vi "V3test.vi"() -> ()   [LabVIEW 2019]
uses:
  WSCbot_V3_Toolkit.lvlibp/WSCBOTV3_Toolkit/Sensor/LowLevel/IR_Chanel.ctl
  WSCbot_V3_Toolkit.lvlibp/WSCBOTV3_Toolkit/MotorControl/LowLevel/ZRaxisRotatingSet.vi
  WSCbot_V3_Toolkit.lvlibp/WSCBOTV3_Toolkit/MotorControl/LowLevel/ZaxisSlideSet.vi
  WSCbot_V3_Toolkit.lvlibp/WSCBOTV3_Toolkit/Sensor/LowLevel/InfraredRanging(Array).vi
  WSCbot_V3_Toolkit.lvlibp
panel:
  in  "?":T1(tab)
  out "EMS":bool
  in  "蜂鳴器":bool
  out "步進馬達旋轉歸零":bool
  out "步進馬達上下歸零":bool
  in  "LED":bool
  in  "旋轉測試":bool
  in  "上下測試":bool
  in  "Enable_R":bool=TRUE
  in  "Enable_L":bool=TRUE
  out "Distance_L(mm)":dbl
  out "Distance_R(mm)":dbl
  out "Valtage":dbl[](array[numeric])
  in  "IR_Chanel":T2[](array[typedef])
  out "R":dbl(graph)
  out "L":dbl(graph)
  in  "Wheel":u16(ring) items=["127mm", "150mm", "100mm"]
  in  "底盤馬達測試":bool
  in  "Speed/ACC":cluster{dbl, dbl}={1000.0, 1000.0}
  in  "XYZ":cluster{"X":dbl, "Y":dbl, "Z":dbl}[](array[cluster])=[{"X"=0.0, "Y"=0.0, "Z"=0.0}]
  in  "Enable?":bool=TRUE
  in  "底盤馬達測試":bool
  in  "4xMotor(deg/s)":dbl[](array[numeric])=[0.0, 0.0, 0.0, 0.0]
  out "ENC (deg)":dbl[](array[numeric])
  out "ENC (deg)":dbl[](array[numeric])
  in  "Stop Button":bool
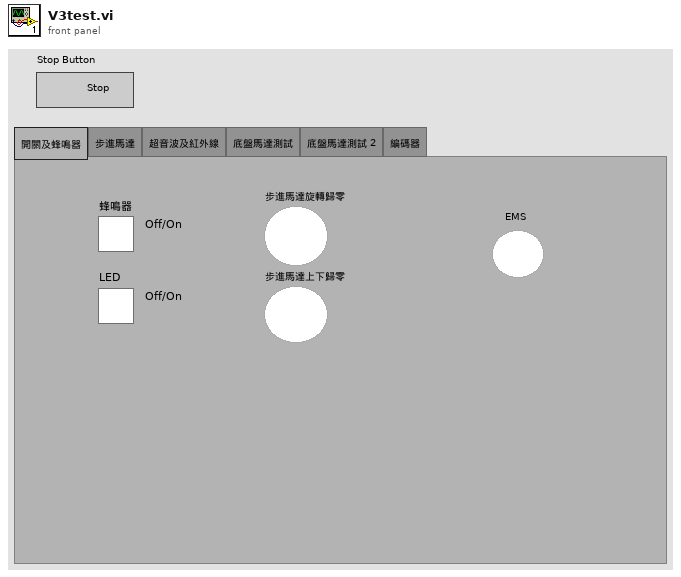
[diagram p1: front panel]
types:
  T1 = enum32{"開關及蜂鳴器", "步進馬達", "超音波及紅外線", "底盤馬達測試", "底盤馬達測試 2", "編碼器"}
  T2 = typedef "WSCbot_V3_Toolkit.lvlibp/IR_Chanel.ctl" = enum16{"IR_LF", "IR_LB", "IR_BL", "IR_BR", "IR_RB", "IR_RF", "IR_FR", "IR_FL"}
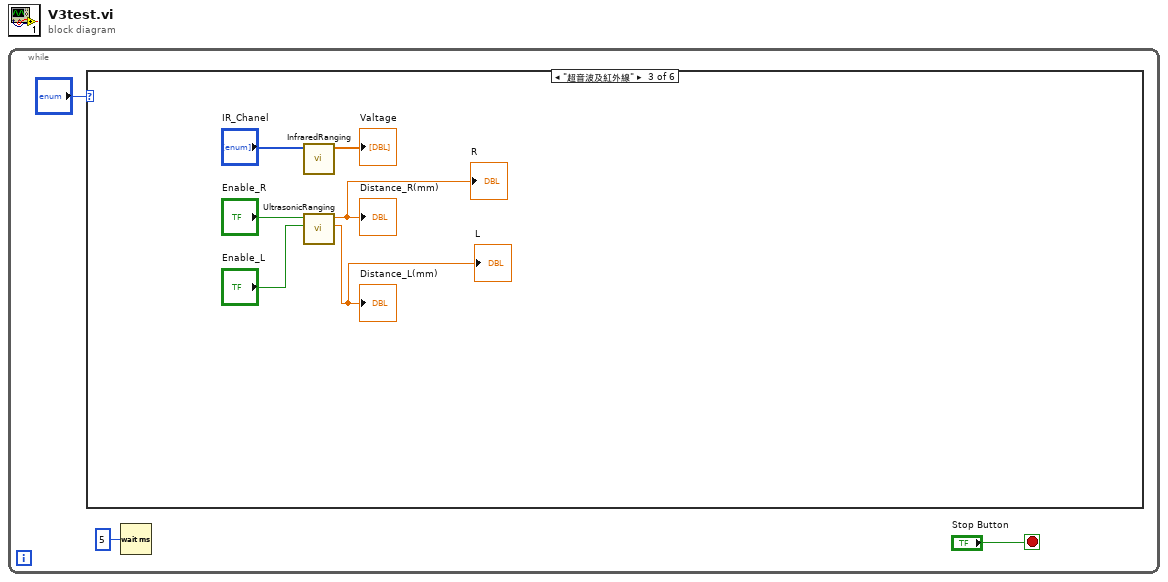
[diagram p0: block diagram]
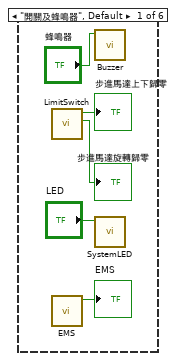
[diagram p2: hidden frame]
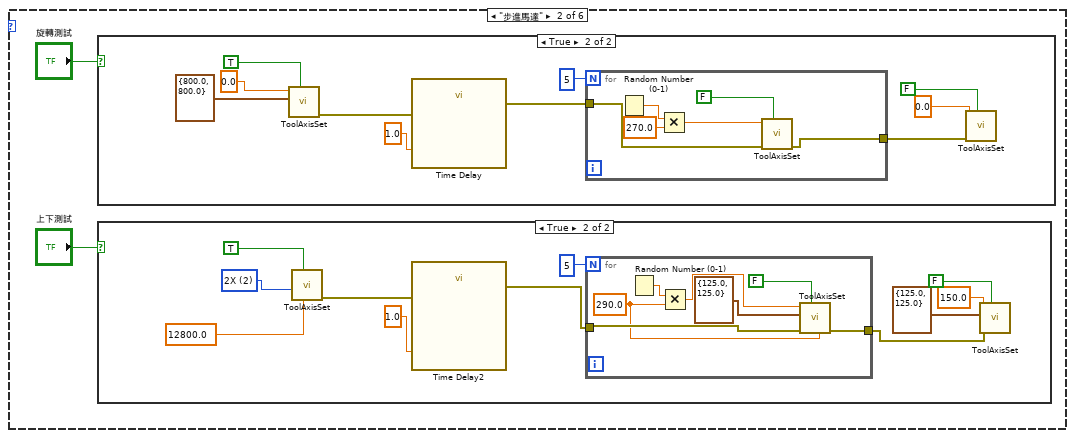
[diagram p3: hidden frame]
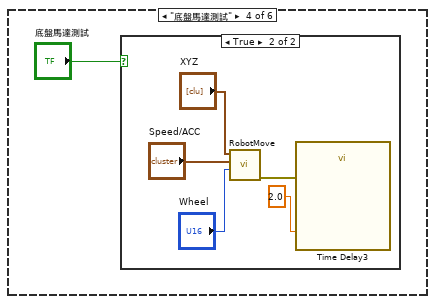
[diagram p6: hidden frame]
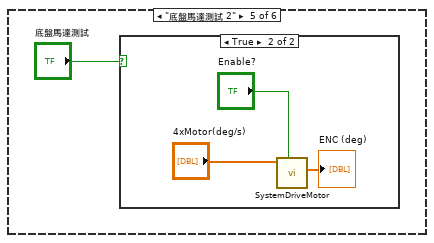
[diagram p8: hidden frame]
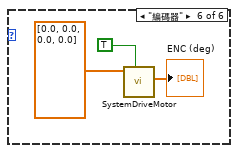
[diagram p10: hidden frame]
diagram:
  n1 = while {
    stop <- "Stop Button" stop-if-true
    n2 = case shown="\"超音波及紅外線\"" "?" {
      frame "開關及蜂鳴器", Default {
        n3 = call "LimitSwitch.vi"() -> ("LS11_ZR_IN"=→"步進馬達旋轉歸零":bool, "LS11_Z_IN"=→"步進馬達上下歸零":bool)  [unwired: 9 in, 1 out]
        n4 = call "EMS.vi"() -> ("EMS"=→"EMS":bool)  [unwired: 10 in, 1 out]
        n5 = call "Buzzer.vi"("Set"="蜂鳴器") -> ()  [unwired: 10 in, 1 out]
        n6 = call "SystemLED.vi"("Set"="LED") -> ()  [unwired: 10 in, 1 out]
      }
      frame "步進馬達" {
        n7 = case shown="True" "旋轉測試" {
          frame False {
          }
          frame True {
            n8 = call-poly "ToolAxisSet.vi"("Reset"=TRUE, "Velocity(deg/s)&ACC(deg/ss)"=cluster{"Velocity(cm/s)":dbl, "ACC(cm/ss)":dbl} {"Velocity(cm/s)"=800.0, "ACC(cm/ss)"=800.0}, "TargetHight(deg)"=0.0) -> ("error out"=w36:errorcluster)  [unwired: 7 in, 1 out]
            n9 = call "Time Delay"("error in (no error)"=w36, "Delay Time (s)"=1.0) -> ("error out"=w35:errorcluster)  [unwired: 9 in]
            n10 = for {
              N: 5 -> [_]
              tunnel: w35 -> [w43]
              tunnel: [w39] -> w30
              n11 = Random Number (0-1)() -> (number: 0 to 1=w42:dbl)
              n12 = Multiply(x=w42, y=270.0) -> (x*y=w41:dbl)
              n13 = call-poly "ToolAxisSet.vi"("Reset"=FALSE, "error in"=w43, "TargetHight(deg)"=w41) -> ("error out"=w39:errorcluster)  [unwired: 7 in, 1 out]
            }
            n14 = call-poly "ToolAxisSet.vi"("Reset"=FALSE, "error in"=w30, "TargetHight(deg)"=0.0) -> ()  [unwired: 7 in, 2 out]
          }
        }
        n15 = case shown="True" "上下測試" {
          frame False {
          }
          frame True {
            w20 = u16 2 items=["0X", "1X", "2X", "3X"] ("findHomeVel (times)")
            n16 = call-poly "ToolAxisSet.vi"("Pulse/rev"=12800.0, "Reset"=TRUE, "findHomeVel (times)"=w20) -> ("error out"=w17:errorcluster)  [unwired: 7 in, 1 out]
            n17 = call "Time Delay2"("error in (no error)"=w17, "Delay Time (s)"=1.0) -> ("error out"=w15:errorcluster)  [unwired: 9 in]
            n18 = for {
              N: 5 -> [_]
              tunnel: w15 -> [w27]
              tunnel: [w22] -> w12
              w24 = 290.0 ("upper limit")
              n19 = Random Number (0-1)() -> (number: 0 to 1=w25:dbl)
              n20 = Multiply(x=w25, y=w24) -> (x*y=w23:dbl)
              n21 = call-poly "ToolAxisSet.vi"("upper limit"=w24, "Reset"=FALSE, "error in"=w27, "Velocity(mm/s)&ACC(mm/ss)"=cluster{"Velocity(cm/s)":dbl, "ACC(cm/ss)":dbl} {"Velocity(cm/s)"=125.0, "ACC(cm/ss)"=125.0}, "TargetABSHight(mm)"=w23) -> ("error out"=w22:errorcluster)  [unwired: 5 in, 1 out]
            }
            n22 = call-poly "ToolAxisSet.vi"("Reset"=FALSE, "error in"=w12, "Velocity(mm/s)&ACC(mm/ss)"=cluster{"Velocity(cm/s)":dbl, "ACC(cm/ss)":dbl} {"Velocity(cm/s)"=125.0, "ACC(cm/ss)"=125.0}, "TargetABSHight(mm)"=150.0) -> ()  [unwired: 6 in, 2 out]
          }
        }
      }
      frame "超音波及紅外線" {
        n23 = call-poly "InfraredRanging.vi"("IR_Chanel"="IR_Chanel") -> ("Valtage"=→"Valtage":dbl[])  [unwired: 9 in, 1 out]
        n24 = call "UltrasonicRanging.vi"("Enable_L"="Enable_L", "Enable_R"="Enable_R") -> ("Distance_L(mm)"=→"Distance_L(mm)" →"L":dbl, "Distance_R(mm)"=→"Distance_R(mm)" →"R":dbl)  [unwired: 7 in, 1 out]
      }
      frame "底盤馬達測試" {
        n25 = case shown="True" "底盤馬達測試" {
          frame False {
          }
          frame True {
            n26 = call "RobotMove.vi"("Wheel"="Wheel", "Speed/ACC"="Speed/ACC", "XYZ"="XYZ") -> ("error out"=w54:errorcluster)  [unwired: 8 in]
            n27 = call "Time Delay3"("error in (no error)"=w54, "Delay Time (s)"=2.0) -> ()  [unwired: 9 in, 1 out]
          }
        }
      }
      frame "底盤馬達測試 2" {
        n28 = case shown="True" "底盤馬達測試" {
          frame False {
          }
          frame True {
            n29 = call "SystemDriveMotor.vi"("Enable?"="Enable?", "4xMotor(deg/s)"="4xMotor(deg/s)") -> ("ENC (deg)"=→"ENC (deg)":dbl[])  [unwired: 8 in, 1 out]
          }
        }
      }
      frame "編碼器" {
        n30 = call "SystemDriveMotor.vi"("Enable?"=TRUE, "4xMotor(deg/s)"=dbl[] [0.0, 0.0, 0.0, 0.0]) -> ("ENC (deg)"=→"ENC (deg)":dbl[])  [unwired: 8 in, 1 out]
      }
    }
    n31 = Wait (ms)(milliseconds to wait=u32 5) -> ()  [unwired: 1 out]
  }
